vi "Read_data.vi"(8 "error in (no error)":errorcluster, 10 "#image":i32, 11 "HIS IN":refnum<class "HIS.lvclass">) -> (0 "error out":errorcluster, 3 "HIS OUT":refnum<class "HIS.lvclass">)   [LabVIEW 2018, in "HIS.lvclass"]
uses:
  HIS.lvclass
  C:/Users/Sergey Denisov/Documents/REPS/TRANCON/Classes/DATA/DATA.lvclass
  DATA.lvclass/DATA.ctl
  HIS.lvclass/HIS.ctl
  DATA.lvclass
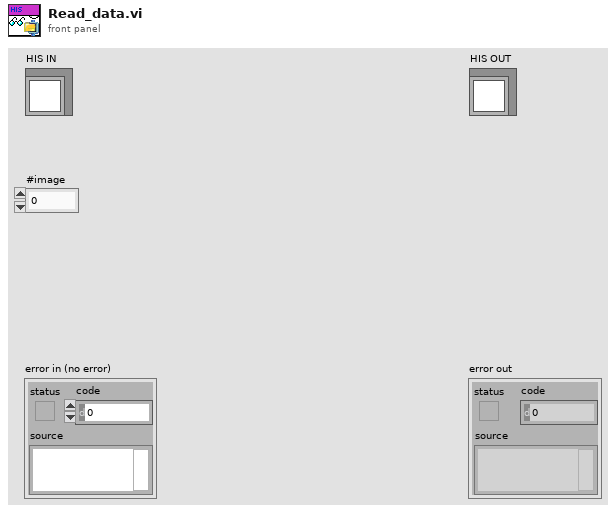
[diagram p1: front panel]
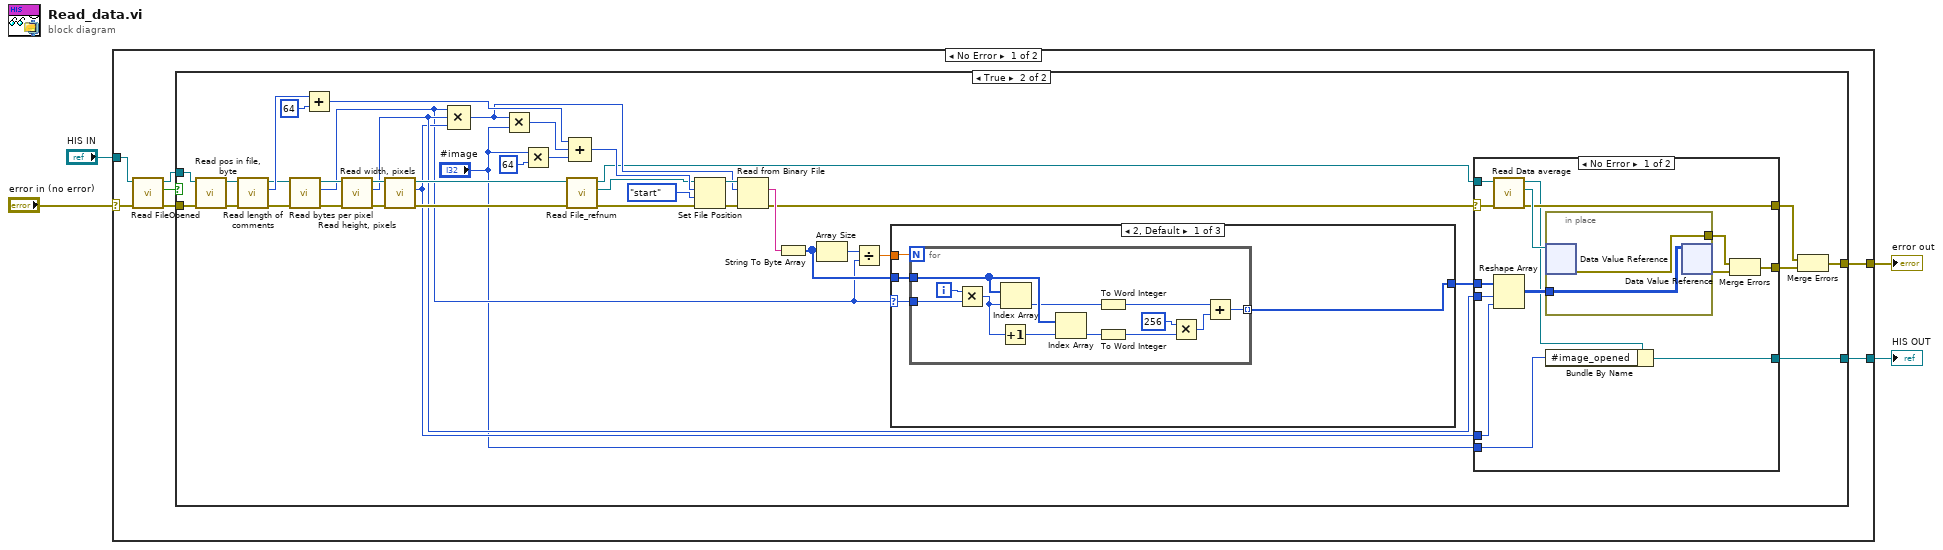
[diagram p0: block diagram]
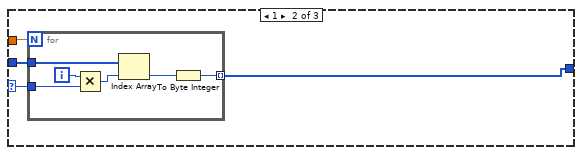
[diagram p4: hidden frame]
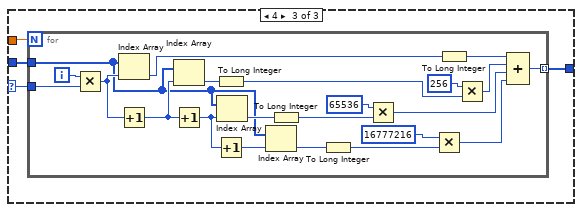
[diagram p5: hidden frame]
diagram:
  n1 = case shown="No Error" "error in (no error)" {
    selector: "error in (no error)" -> [w11 w125]
    tunnel: [w5 w125] -> w3
    tunnel: [w8 w124] -> w2
    tunnel: "HIS IN" -> [w10 w124]
    frame No Error {
      n2 = call "Read FileOpened.vi"("error in (no error)"=w11, "DATA in"=w10) -> ("error out"=w6:errorcluster, "FileOpened"=w9:bool, "DATA out"=w7:refnum<class "HIS.lvclass">)  [unwired: 7 in]
      n3 = case shown="True" w9 {
        tunnel: [w13 w22] -> w8
        tunnel: w7 -> [w13 w50]
        tunnel: w6 -> [w12 w51]
        tunnel: [w12 w20] -> w5
        frame False {
        }
        frame True {
          n4 = call "Read pos in file, byte.vi"("error in (no error)"=w51, "DATA in"=w50) -> ("error out"=w47:errorcluster, "DATA out"=w45:refnum<class "HIS.lvclass">)  [unwired: 7 in, 1 out]
          n5 = call "Read length of comments.vi"("error in (no error)"=w47, "DATA in"=w45) -> ("error out"=w46:errorcluster, "length of comments"=w53:i32, "DATA out"=w44:refnum<class "HIS.lvclass">)  [unwired: 7 in]
          n6 = call "Read bytes per pixel.vi"("error in (no error)"=w46, "DATA in"=w44) -> ("error out"=w49:errorcluster, "bytes per pixel"=w17:i8, "DATA out"=w43:refnum<class "HIS.lvclass">)  [unwired: 7 in]
          n7 = Add(x=w53, y=64) -> (x+y=w40:i32)
          n8 = call "Read height, pixels.vi"("error in (no error)"=w49, "DATA in"=w43) -> ("error out"=w48:errorcluster, "height, pixels"=w19:i32, "DATA out"=w42:refnum<class "HIS.lvclass">)  [unwired: 7 in]
          n9 = call "Read width, pixels.vi"("error in (no error)"=w48, "DATA in"=w42) -> ("error out"=w35:errorcluster, "width, pixels"=w18:i32, "DATA out"=w33:refnum<class "HIS.lvclass">)  [unwired: 7 in]
          n10 = Compound Arithmetic op=MULTIPLY(w17, w19, w18) -> (w24:i32)
          n11 = Multiply(x=w24, y="#image") -> (x*y=w39:i32)
          n12 = Multiply(x="#image", y=64) -> (x*y=w38:i32)
          n13 = call "Read File_refnum.vi"("error in (no error)"=w35, "DATA in"=w33) -> ("error out"=w32:errorcluster, "File_refnum"=w34:refnum<file>, "DATA out"=w23:refnum<class "HIS.lvclass">)  [unwired: 7 in]
          n14 = Compound Arithmetic op=ADD(w40, w39, w38) -> (w37:i32)
          n15 = Set File Position(offset (in bytes) (0)=w37, refnum=w34, from (0:start)=enum16{"start", "end", "current"}."start", error in=w32) -> (refnum out=w26:refnum<file>, error out=w25:errorcluster)
          n16 = Read from Binary File(8:w25, 10:w24, 11:w26) -> (0:w16:errorcluster, 2:w27:string)  [unwired: 5 out]
          n17 = String To Byte Array(string=w27) -> (unsigned byte array=w31:u8[])
          n18 = Array Size(array=w31) -> (size(s)=w30:i32)
          n19 = Divide(x=w30, y=w17) -> (x/y=w29:dbl)
          n20 = case shown="2, Default" w17 {
            selector: w17 -> [w73 w89 w101]
            tunnel: w31 -> [w74 w90 w100]
            tunnel: w29 -> [w75 w91 w99]
            tunnel: [w72 w88 w98] -> w28
            frame 2, Default {
              n21 = for {
                N: w75 -> [_]
                tunnel: w74 -> [w85]
                tunnel: [w78] -> w72 mode=indexing
                tunnel: w73 -> [w86]
                i -> [w87]
                n22 = Multiply(x=w87, y=w86) -> (x*y=w84:i32)
                n23 = Increment(x=w84) -> (x+1=w83:i32)
                n24 = Index Array(array=w85, index=w84) -> (element=w80:u8)
                n25 = Index Array(array=w85, index=w83) -> (element=w82:u8)
                n26 = To Word Integer(number=w80) -> (16bit integer=w76:i16)
                n27 = To Word Integer(number=w82) -> (16bit integer=w77:i16)
                n28 = Multiply(x=i16 256, y=w77) -> (x*y=w79:i16)
                n29 = Add(x=w76, y=w79) -> (x+y=w78:i16)
              }
            }
            frame 1 {
              n30 = for {
                N: w91 -> [_]
                tunnel: w90 -> [w95]
                tunnel: [w92] -> w88 mode=indexing
                tunnel: w89 -> [w96]
                i -> [w97]
                n31 = Multiply(x=w97, y=w96) -> (x*y=w94:i32)
                n32 = Index Array(array=w95, index=w94) -> (element=w93:u8)
                n33 = To Byte Integer(number=w93) -> (8bit integer=w92:i8)
              }
            }
            frame 4 {
              n34 = for {
                N: w99 -> [_]
                tunnel: w100 -> [w108]
                tunnel: w101 -> [w102]
                tunnel: [w118] -> w98 mode=indexing
                i -> [w123]
                n35 = Multiply(x=w123, y=w102) -> (x*y=w122:i32)
                n36 = Index Array(array=w108, index=w122) -> (element=w120:u8)
                n37 = Increment(x=w122) -> (x+1=w117:i32)
                n38 = Index Array(array=w108, index=w117) -> (element=w113:u8)
                n39 = Increment(x=w117) -> (x+1=w109:i32)
                n40 = To Long Integer(number=w113) -> (32bit integer=w112:i32)
                n41 = Increment(x=w109) -> (x+1=w107:i32)
                n42 = Index Array(array=w108, index=w109) -> (element=w116:u8)
                n43 = Index Array(array=w108, index=w107) -> (element=w106:u8)
                n44 = To Long Integer(number=w116) -> (32bit integer=w111:i32)
                n45 = To Long Integer(number=w106) -> (32bit integer=w105:i32)
                n46 = Multiply(x=65536, y=w111) -> (x*y=w110:i32)
                n47 = Multiply(x=16777216 ("y"), y=w105) -> (x*y=w104:i32)
                n48 = To Long Integer(number=w120) -> (32bit integer=w114:i32)
                n49 = Multiply(x=i16 256, y=w112) -> (x*y=w119:i32)
                n50 = Compound Arithmetic op=ADD(w114, w119, w110, w104) -> (w118:i32)
              }
            }
          }
          n51 = case shown="No Error" w16 {
            selector: w16 -> [w60 w70]
            tunnel: w28 -> [w67 _]
            tunnel: w23 -> [w65 w71]
            tunnel: [w55 w71] -> w22
            tunnel: [w63 w70] -> w21
            tunnel: w19 -> [w62 _]
            tunnel: w18 -> [w61 _]
            tunnel: [w57 _] -> w15
            tunnel: "#image" -> [w54 _]
            frame No Error {
              n52 = call "Read Data average.vi"("error in (no error)"=w60, "DATA in"=w65) -> ("error out"=w63:errorcluster, "Data average"=w66:refnum<data-value>, "DATA out"=w56:refnum<class "HIS.lvclass">)  [unwired: 7 in]
              n53 = Reshape Array(w67, w62, w61) -> (w64:i32[][])
              n54 = in-place {
                in-place-border: w64 -> [w69]
                in-place-border: [w68] -> w59
                n55 = in-place-dvr #1(w66) -> (w68:errorcluster)  [unwired: 1 out]
                n56 = in-place-dvr #1(w69) -> (w58:errorcluster)  [unwired: 1 out]
              }
              n57 = Bundle By Name(cluster=w56, "#image_opened"=w54) -> (w55:refnum<class "HIS.lvclass">)
              n58 = Merge Errors(w59, w58) -> (w57:errorcluster)
            }
            frame Error {
            }
          }
          n59 = Merge Errors(w21, w15) -> (w20:errorcluster)
        }
      }
    }
    frame Error {
    }
  }
  "error out" <- w3
  "HIS OUT" <- w2
